vi "TestStand_Control ( Process_XML ).vi"(8 "error in":errorcluster, 11 "file path (use dialog)":path) -> (0 "error out":errorcluster)   [LabVIEW 2018, in "TestStand_Control.lvlib"]
uses:
  TestStand_Control.lvlib
panel:
  out "result string":string
  out "text":string
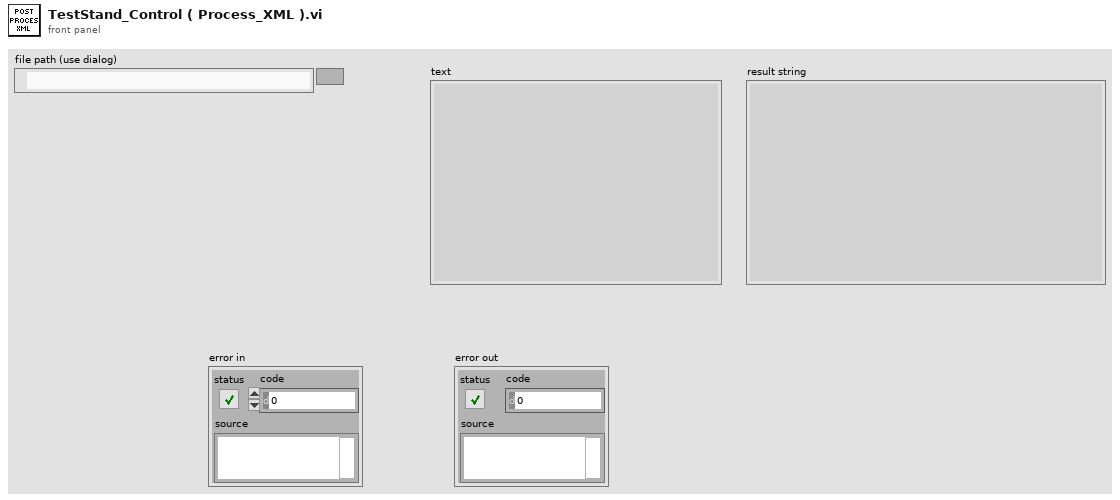
[diagram p1: front panel]
types:
  T1 = enum16{"open", "replace", "create", "open or create", "replace or create", "replace or create with confirmation"}
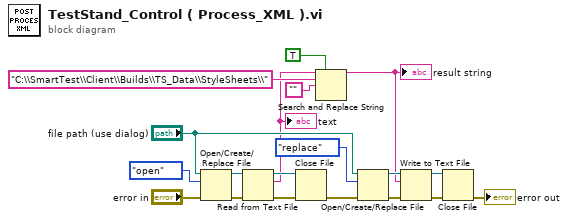
[diagram p0: block diagram]
diagram:
  n1 = Open/Create/Replace File(file path (use dialog)="file path (use dialog)", error in="error in", operation (0:open)=T1."open") -> (refnum out=w19:refnum<file>, error out=w13:errorcluster)  [unwired: 3 in, 1 out]
  n2 = Read from Text File(file (use dialog)=w19, error in=w13) -> (refnum out=w14:refnum<file>, text=w4:string, error out=w12:errorcluster)  [unwired: 2 in, 1 out]
  "text" <- w4
  n3 = Close File(refnum=w14, error in=w12) -> (error out=w9:errorcluster)  [unwired: 1 out]
  n4 = Search and Replace String(replace all?=TRUE ("replace all? (F)"), input string=w4, search string="C:\\SmartTest\\Client\\Builds\\TS_Data\\StyleSheets\\" ("input string"), replace string="" ("search string")) -> (result string=w5:string)  [unwired: 4 in, 3 out]
  "result string" <- w5
  n5 = Open/Create/Replace File(file path (use dialog)="file path (use dialog)", error in=w9, operation (0:open)=T1."replace") -> (refnum out=w7:refnum<file>, error out=w6:errorcluster)  [unwired: 3 in, 1 out]
  n6 = Write to Text File(file (use dialog)=w7, text=w5, error in=w6) -> (refnum out=w3:refnum<file>, error out=w2:errorcluster)  [unwired: 1 in, 1 out]
  n7 = Close File(refnum=w3, error in=w2) -> (error out=→"error out":errorcluster)  [unwired: 1 out]
